vi "TLMB Config Parse.vi"(0 "Config File Path":path=path "C:/Automation/Configurations/VALEW.config", 11 "Error In":errorcluster) -> (4 "Pass/Fail?":bool, 6 "Report Text":string, 8 "TLMB_config":T1, 15 "Error Out":errorcluster)   [LabVIEW 2018, in "TLMB.lvlib"]
doc: "Opens a reference and set the initial configuration coming from the File TLMB.confg."
uses:
  Projects/TLMB.lvlib
  type defs/TLMB Config.ctl
  <vilib>/Utility/config.llb/Read Key (String).vi
  <vilib>/Utility/config.llb/Read Key (Boolean).vi
  <vilib>/Utility/config.llb/NI_LVConfig.lvlib
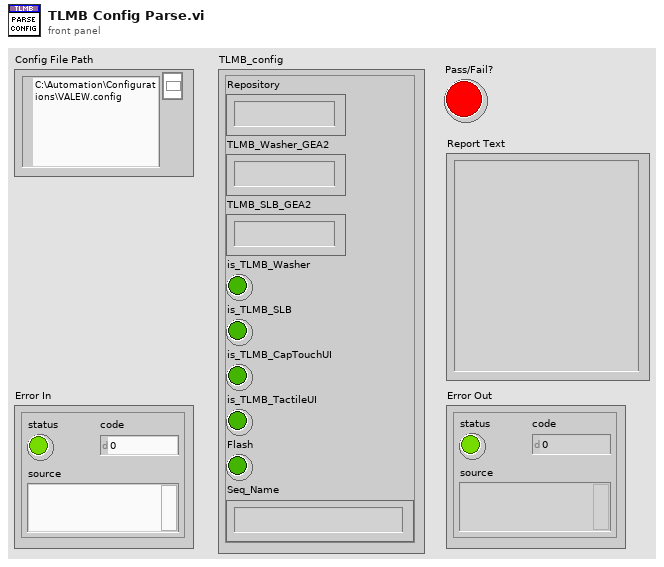
[diagram p1: front panel]
types:
  T1 = typedef "TLMB.lvlib/TLMB Config.ctl" = cluster{"Repository":string, "TLMB_Washer_GEA2":string, "TLMB_SLB_GEA2":string, "is_TLMB_Washer":bool, "is_TLMB_SLB":bool, "is_TLMB_CapTouchUI":bool, "is_TLMB_TactileUI":bool, "Flash":bool, "Seq_Name":string}
  T2 = typedef "NI_LVConfig.lvlib/Config Data RefNum.ctl" = refnum<k1>
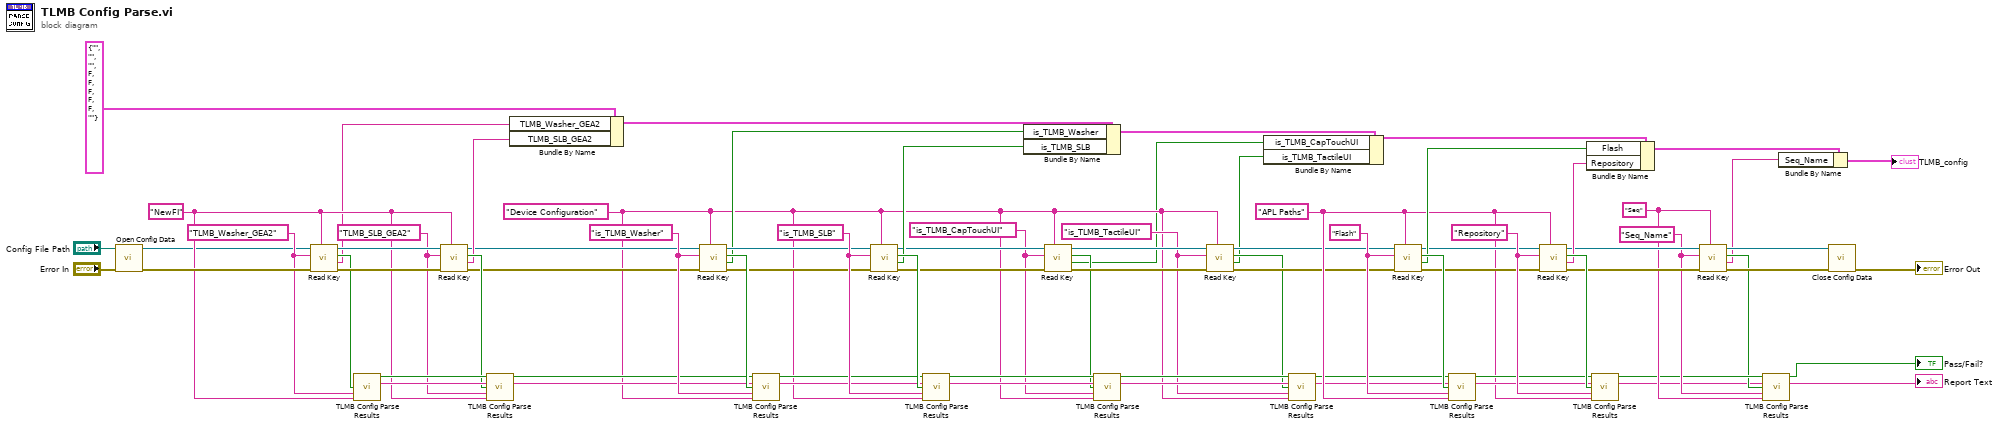
[diagram p0: block diagram]
diagram:
  w5 = "is_TLMB_TactileUI" ("key")
  w9 = "is_TLMB_CapTouchUI" ("key")
  w42 = "Seq_Name" ("key")
  w41 = "Seq" ("section")
  w54 = "Repository" ("key")
  w62 = "is_TLMB_SLB" ("key")
  w64 = "Flash" ("key")
  w38 = "APL Paths" ("section")
  w66 = "is_TLMB_Washer" ("key")
  w4 = "Device Configuration" ("section")
  w68 = "TLMB_SLB_GEA2" ("key")
  w73 = "TLMB_Washer_GEA2" ("key")
  w63 = "NewFI" ("section")
  n1 = call <vilib>:"Open Config Data.vi"("error in (no error)"="Error In", "configuration file path"="Config File Path") -> ("error out"=w76:errorcluster, "refnum"=w47:T2)  [unwired: 7 in, 1 out]
  n2 = call-poly <vilib>:"Read Key.vi"("section"=w63, "error in (no error)"=w76, "key"=w73, "refnum"=w47) -> ("error out"=w77:errorcluster, "value"=w29:string, "found?"=w72:bool, "refnum out"=w78:T2)  [unwired: 4 in]
  n3 = call "TLMB Config Parse Results.vi"("found?"=w72, "key"=w73, "section"=w63) -> ("Pass/Fail"=w71:bool, "Report Text"=w70:string)  [unwired: 11 in]
  n4 = call-poly <vilib>:"Read Key.vi"("section"=w63, "error in (no error)"=w77, "key"=w68, "refnum"=w78) -> ("error out"=w23:errorcluster, "value"=w30:string, "found?"=w69:bool, "refnum out"=w24:T2)  [unwired: 4 in]
  n5 = call "TLMB Config Parse Results.vi"("Previous Pass/Fail"=w71, "Previous Report Text"=w70, "found?"=w69, "key"=w68, "section"=w63) -> ("Pass/Fail"=w27:bool, "Report Text"=w28:string)  [unwired: 9 in]
  n6 = Bundle By Name(cluster=T1 {"Repository"="", "TLMB_Washer_GEA2"="", "TLMB_SLB_GEA2"="", "is_TLMB_Washer"=FALSE, "is_TLMB_SLB"=FALSE, "is_TLMB_CapTouchUI"=FALSE, "is_TLMB_TactileUI"=FALSE, "Flash"=FALSE, "Seq_Name"=""} ("VALEW_config"), "TLMB_Washer_GEA2"=w29, "TLMB_SLB_GEA2"=w30) -> (w26:T1)
  n7 = call-poly <vilib>:"Read Key.vi"("section"=w4, "error in (no error)"=w23, "key"=w66, "refnum"=w24) -> ("error out"=w59:errorcluster, "value"=w25:bool, "found?"=w67:bool, "refnum out"=w60:T2)  [unwired: 4 in]
  n8 = call "TLMB Config Parse Results.vi"("Previous Pass/Fail"=w27, "Previous Report Text"=w28, "found?"=w67, "key"=w66, "section"=w4) -> ("Pass/Fail"=w58:bool, "Report Text"=w57:string)  [unwired: 9 in]
  n9 = call-poly <vilib>:"Read Key.vi"("section"=w4, "error in (no error)"=w59, "key"=w62, "refnum"=w60) -> ("error out"=w21:errorcluster, "value"=w22:bool, "found?"=w61:bool, "refnum out"=w18:T2)  [unwired: 4 in]
  n10 = call "TLMB Config Parse Results.vi"("Previous Pass/Fail"=w58, "Previous Report Text"=w57, "found?"=w61, "key"=w62, "section"=w4) -> ("Pass/Fail"=w15:bool, "Report Text"=w12:string)  [unwired: 9 in]
  n11 = Bundle By Name(cluster=w26, "is_TLMB_Washer"=w25, "is_TLMB_SLB"=w22) -> (w7:T1)
  n12 = call-poly <vilib>:"Read Key.vi"("section"=w4, "error in (no error)"=w21, "key"=w9, "refnum"=w18) -> ("error out"=w20:errorcluster, "value"=w2:bool, "found?"=w8:bool, "refnum out"=w17:T2)  [unwired: 4 in]
  n13 = call "TLMB Config Parse Results.vi"("Previous Pass/Fail"=w15, "Previous Report Text"=w12, "found?"=w8, "key"=w9, "section"=w4) -> ("Pass/Fail"=w14:bool, "Report Text"=w11:string)  [unwired: 9 in]
  n14 = call-poly <vilib>:"Read Key.vi"("section"=w4, "error in (no error)"=w20, "key"=w5, "refnum"=w17) -> ("error out"=w19:errorcluster, "value"=w1:bool, "found?"=w3:bool, "refnum out"=w16:T2)  [unwired: 4 in]
  n15 = Bundle By Name(cluster=w7, "is_TLMB_CapTouchUI"=w2, "is_TLMB_TactileUI"=w1) -> (w6:T1)
  n16 = call "TLMB Config Parse Results.vi"("Previous Pass/Fail"=w14, "Previous Report Text"=w11, "found?"=w3, "key"=w5, "section"=w4) -> ("Pass/Fail"=w13:bool, "Report Text"=w10:string)  [unwired: 9 in]
  n17 = call-poly <vilib>:"Read Key.vi"("section"=w38, "error in (no error)"=w19, "key"=w64, "refnum"=w16) -> ("error out"=w49:errorcluster, "value"=w56:bool, "found?"=w65:bool, "refnum out"=w50:T2)  [unwired: 4 in]
  n18 = call "TLMB Config Parse Results.vi"("Previous Pass/Fail"=w13, "Previous Report Text"=w10, "found?"=w65, "key"=w64, "section"=w38) -> ("Pass/Fail"=w52:bool, "Report Text"=w51:string)  [unwired: 9 in]
  n19 = call-poly <vilib>:"Read Key.vi"("section"=w38, "error in (no error)"=w49, "key"=w54, "refnum"=w50) -> ("error out"=w46:errorcluster, "value"=w48:string, "found?"=w55:bool, "refnum out"=w44:T2)  [unwired: 4 in]
  n20 = Bundle By Name(cluster=w6, "Flash"=w56, "Repository"=w48) -> (w37:T1)
  n21 = call "TLMB Config Parse Results.vi"("Previous Pass/Fail"=w52, "Previous Report Text"=w51, "found?"=w55, "key"=w54, "section"=w38) -> ("Pass/Fail"=w40:bool, "Report Text"=w32:string)  [unwired: 9 in]
  n22 = call-poly <vilib>:"Read Key.vi"("section"=w41, "error in (no error)"=w46, "key"=w42, "refnum"=w44) -> ("error out"=w45:errorcluster, "value"=w36:string, "found?"=w39:bool, "refnum out"=w43:T2)  [unwired: 4 in]
  n23 = call "TLMB Config Parse Results.vi"("Previous Pass/Fail"=w40, "Previous Report Text"=w32, "found?"=w39, "key"=w42, "section"=w41) -> ("Pass/Fail"=→"Pass/Fail?":bool, "Report Text"=→"Report Text":string)  [unwired: 9 in]
  n24 = Bundle By Name(cluster=w37, "Seq_Name"=w36) -> (→"TLMB_config":T1)
  n25 = call <vilib>:"Close Config Data.vi"("error in (no error)"=w45, "refnum"=w43) -> ("error out"=→"Error Out":errorcluster)  [unwired: 8 in, 1 out]
